vi "__GetStatsLadder.vi"(8 "error in (no error)":errorcluster, 11 "ClashRoyale in":refnum<class "ClashRoyale.lvclass">) -> (0 "error out":errorcluster, 3 "ClashRoyale out":refnum<class "ClashRoyale.lvclass">)   [LabVIEW 2020, in "ClashRoyale.lvclass"]
uses:
  ClashRoyale.lvclass
  ClashRoyale.lvclass/ClashRoyale.ctl
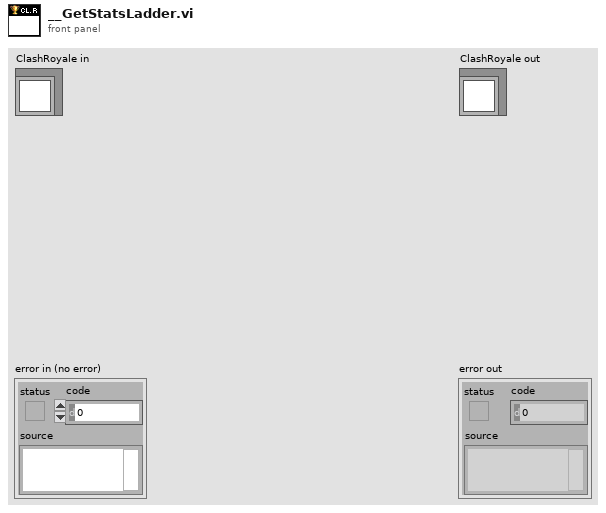
[diagram p1: front panel]
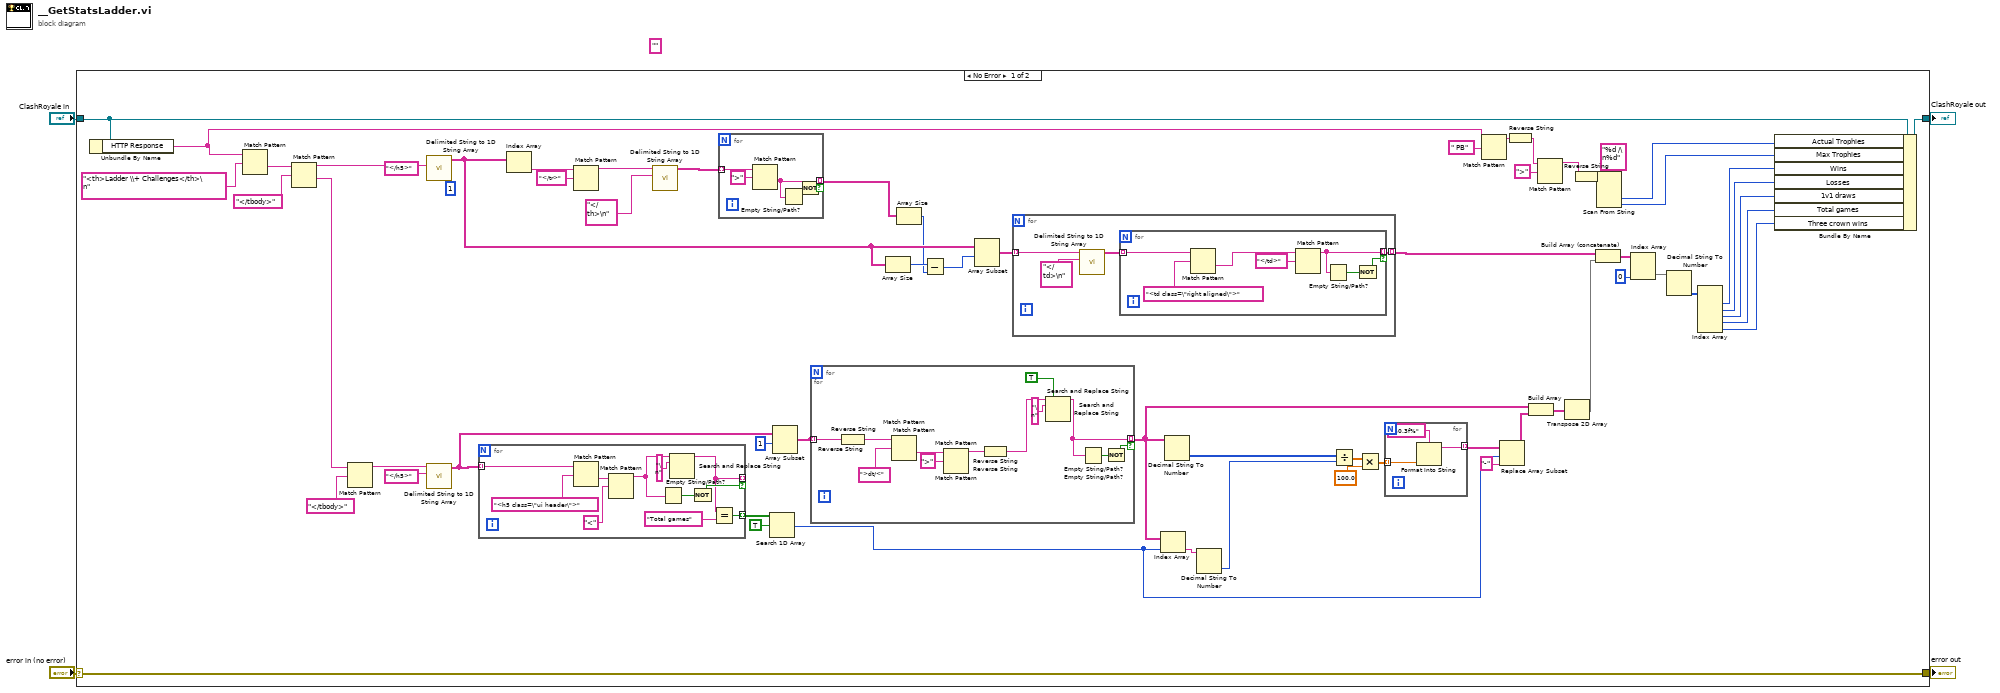
[diagram p0: block diagram]
diagram:
  (unwired) ""
  n1 = case shown="No Error" "error in (no error)" {
    selector: "error in (no error)" -> [w65 w121]
    tunnel: [w65 w121] -> w3
    tunnel: [w24 w120] -> w1
    tunnel: "ClashRoyale in" -> [w25 w120]
    frame No Error {
      (unwired) 1 ("index")
      n2 = Unbundle By Name(w25) -> ("HTTP Response"=w5:string)
      n3 = Match Pattern(string=w5, regular expression="<th>Ladder \\+ Challenges</th>\n") -> (after substring=w60:string)  [unwired: 1 in, 3 out]
      n4 = Match Pattern(string=w60, regular expression="</tbody>") -> (before substring=w57:string, after substring=w48:string)  [unwired: 1 in, 2 out]
      n5 = Match Pattern(string=w48, regular expression="</tbody>") -> (before substring=w51:string)  [unwired: 1 in, 3 out]
      n6 = call <vilib>:"Delimited String to 1D String Array.vi"("delimiter"="</h5>", "delimited string"=w57) -> ("string array"=w55:string[])  [unwired: 9 in]
      n7 = call <vilib>:"Delimited String to 1D String Array.vi"("delimiter"="</h5>", "delimited string"=w51) -> ("string array"=w47:string[])  [unwired: 9 in]
      n8 = for {
        tunnel: w47 -> [w102] mode=indexing
        tunnel: [w95] -> _ mode=indexing if=w100
        tunnel: [w93] -> w34 mode=indexing
        n9 = Match Pattern(string=w102, regular expression="<h5 class=\"ui header\">") -> (after substring=w99:string)  [unwired: 1 in, 3 out]
        n10 = Match Pattern(string=w99, regular expression="<") -> (before substring=w97:string)  [unwired: 1 in, 3 out]
        n11 = Empty String/Path?(string/path=w97) -> (empty?=w101:bool)
        n12 = Search and Replace String(input string=w97, search string="\n") -> (result string=w95:string)  [unwired: 6 in, 3 out]
        n13 = Not(x=w101) -> (.not. x?=w100:bool)
        n14 = Equal?(x=w95, y="Total games") -> (x = y?=w93:bool)
      }
      n15 = Index Array(array=w55) -> (element=w56:string)  [unwired: 1 in]
      n16 = Match Pattern(string=w56, regular expression="</tr>") -> (before substring=w62:string)  [unwired: 1 in, 3 out]
      n17 = call <vilib>:"Delimited String to 1D String Array.vi"("delimiter"="</th>\n", "delimited string"=w62) -> ("string array"=w61:string[])  [unwired: 9 in]
      n18 = for {
        tunnel: w61 -> [w119] mode=indexing
        tunnel: [w117] -> w52 mode=indexing if=w115
        n19 = Match Pattern(string=w119, regular expression=">") -> (after substring=w117:string)  [unwired: 1 in, 3 out]
        n20 = Empty String/Path?(string/path=w117) -> (empty?=w116:bool)
        n21 = Not(x=w116) -> (.not. x?=w115:bool)
      }
      n22 = Search 1D Array(1D array=w34, element=TRUE) -> (index of element=w29:i32)  [unwired: 1 in]
      n23 = Array Subset(array=w47, index=1) -> (w27:string[])  [unwired: 1 in]
      n24 = for {
        tunnel: w27 -> [w69] mode=indexing
        tunnel: [w77] -> _ mode=indexing if=w68
        n25 = Reverse String(1:w69) -> (0:w67:string)
        n26 = Match Pattern(string=w67, regular expression=">dt/<") -> (after substring=w74:string)  [unwired: 1 in, 3 out]
        n27 = Match Pattern(string=w74, regular expression=">") -> (before substring=w71:string)  [unwired: 1 in, 3 out]
        n28 = Reverse String(1:w71) -> (0:w66:string)
        n29 = Search and Replace String(replace all?=TRUE ("replace all? (F)"), input string=w66, search string="\n") -> (result string=w77:string)  [unwired: 5 in, 3 out]
        n30 = Empty String/Path?(string/path=w77) -> (empty?=w73:bool)
        n31 = Not(x=w73) -> (.not. x?=w68:bool)
      }
      n32 = for {
        tunnel: w27 -> [w84] mode=indexing
        tunnel: [w92] -> w32 mode=indexing if=w83
        n33 = Reverse String(1:w84) -> (0:w82:string)
        n34 = Match Pattern(string=w82, regular expression=">dt/<") -> (after substring=w89:string)  [unwired: 1 in, 3 out]
        n35 = Match Pattern(string=w89, regular expression=">") -> (before substring=w86:string)  [unwired: 1 in, 3 out]
        n36 = Reverse String(1:w86) -> (0:w81:string)
        n37 = Search and Replace String(replace all?=TRUE ("replace all? (F)"), input string=w81, search string="\n") -> (result string=w92:string)  [unwired: 5 in, 3 out]
        n38 = Empty String/Path?(string/path=w92) -> (empty?=w88:bool)
        n39 = Not(x=w88) -> (.not. x?=w83:bool)
      }
      n40 = Array Size(array=w55) -> (size(s)=w54:i32)
      n41 = Array Size(array=w52) -> (size(s)=w45:i32)
      n42 = Subtract(x=w54, y=w45) -> (x-y=w53:i32)
      n43 = Array Subset(array=w55, index=w53) -> (w26:string[])  [unwired: 1 in]
      n44 = for {
        tunnel: w26 -> [w106] mode=indexing
        tunnel: [w104] -> w43 mode=indexing
        n45 = call <vilib>:"Delimited String to 1D String Array.vi"("delimiter"="</td>\n", "delimited string"=w106) -> ("string array"=w105:string[])  [unwired: 9 in]
        n46 = for {
          tunnel: w105 -> [w111] mode=indexing
          tunnel: [w109] -> w104 mode=indexing if=w108
          n47 = Match Pattern(string=w111, regular expression="<td class=\"right aligned\">") -> (after substring=w112:string)  [unwired: 1 in, 3 out]
          n48 = Match Pattern(string=w112, regular expression="</td>") -> (before substring=w109:string)  [unwired: 1 in, 3 out]
          n49 = Empty String/Path?(string/path=w109) -> (empty?=w110:bool)
          n50 = Not(x=w110) -> (.not. x?=w108:bool)
        }
      }
      n51 = Index Array(array=w32, index=w29) -> (element=w42:string)
      n52 = Decimal String To Number(string=w32) -> (number=w41:i32[])  [unwired: 2 in, 1 out]
      n53 = Decimal String To Number(string=w42) -> (number=w31:i32)  [unwired: 2 in, 1 out]
      n54 = Divide(x=w41, y=w31) -> (x/y=w40:dbl[])
      n55 = Multiply(x=w40, y=100.0) -> (x*y=w38:dbl[])
      n56 = for {
        tunnel: w38 -> [w80] mode=indexing
        tunnel: [w78] -> w37 mode=indexing
        n57 = Format Into String(format string="%0.3f%", w80) -> (resulting string=w78:string)  [unwired: 2 in, 1 out]
      }
      n58 = Match Pattern(string=w5, regular expression=" PB") -> (before substring=w13:string)  [unwired: 1 in, 3 out]
      n59 = Replace Array Subset(array=w37, new element="-" ("new element/subarray"), index=w29) -> (w30:string[])
      n60 = Reverse String(1:w13) -> (0:w10:string)
      n61 = Build Array(w32, w30) -> (w36:string[][])
      n62 = Match Pattern(string=w10, regular expression=">") -> (before substring=w9:string)  [unwired: 1 in, 3 out]
      n63 = Transpose 2D Array(2D array=w36) -> (transposed array=w35:string[][])
      n64 = Reverse String(1:w9) -> (0:w8:string)
      n65 = Build Array (concatenate)(w43, w35) -> (w23:string[][])
      n66 = Scan From String(format string="%d /\n%d", input string=w8) -> (output 1=w7:i32, output 2=w6:i32)  [unwired: 4 in, 3 out]
      n67 = Index Array(array=w23, index (col)=0 ("disabled index (col)")) -> (element=w21:string[])  [unwired: 1 in]
      n68 = Decimal String To Number(string=w21) -> (number=w20:i32[])  [unwired: 2 in, 1 out]
      n69 = Index Array(array=w20) -> (element #1=w19:i32, element #2=w18:i32, element #3=w17:i32, element #4=w16:i32, element #5=w15:i32)  [unwired: 5 in]
      n70 = Bundle By Name(cluster=w25, "Actual Trophies"=w7, "Max Trophies"=w6, "Wins"=w19, "Losses"=w18, "1v1 draws"=w17, "Total games"=w16, "Three crown wins"=w15) -> (w24:refnum<class "ClashRoyale.lvclass">)
    }
    frame Error {
    }
  }
  "error out" <- w3
  "ClashRoyale out" <- w1
